vi "edit sensor.vi"(0 "CalibrationData in":T1, 1 "new":bool, 5 "id":u32) -> (4 "CalibrationData out":T1, 6 "canceled":bool, 8 "row":i32)   [LabVIEW 2019, in "GUI Sensor Lib.lvclass"]
uses:
  GUI Sensor Lib.lvclass
  TypeDef/CalibrationData.ctl
  TypeDef/GUI Setting Channel.ctl
  TypeDef/SensorCalibrationData.ctl
panel:
  in  "Scaled":dbl caption="Калиброванное  значение"
  in  "Raw":dbl caption="Необработанное значение"
  in  "ref channel":i16(ring) caption="Канал" items=["Ввод необработанного зачения вручную"=-1]
  in  "data":i32(listbox)
  in  "Remove":bool
  in  "Add":bool
  out "XY Graph - Dark":cluster{dbl[], dbl[]}[](graph)
  in  "Close":bool
  in  "OK":bool
  in  "name":string caption="Название"
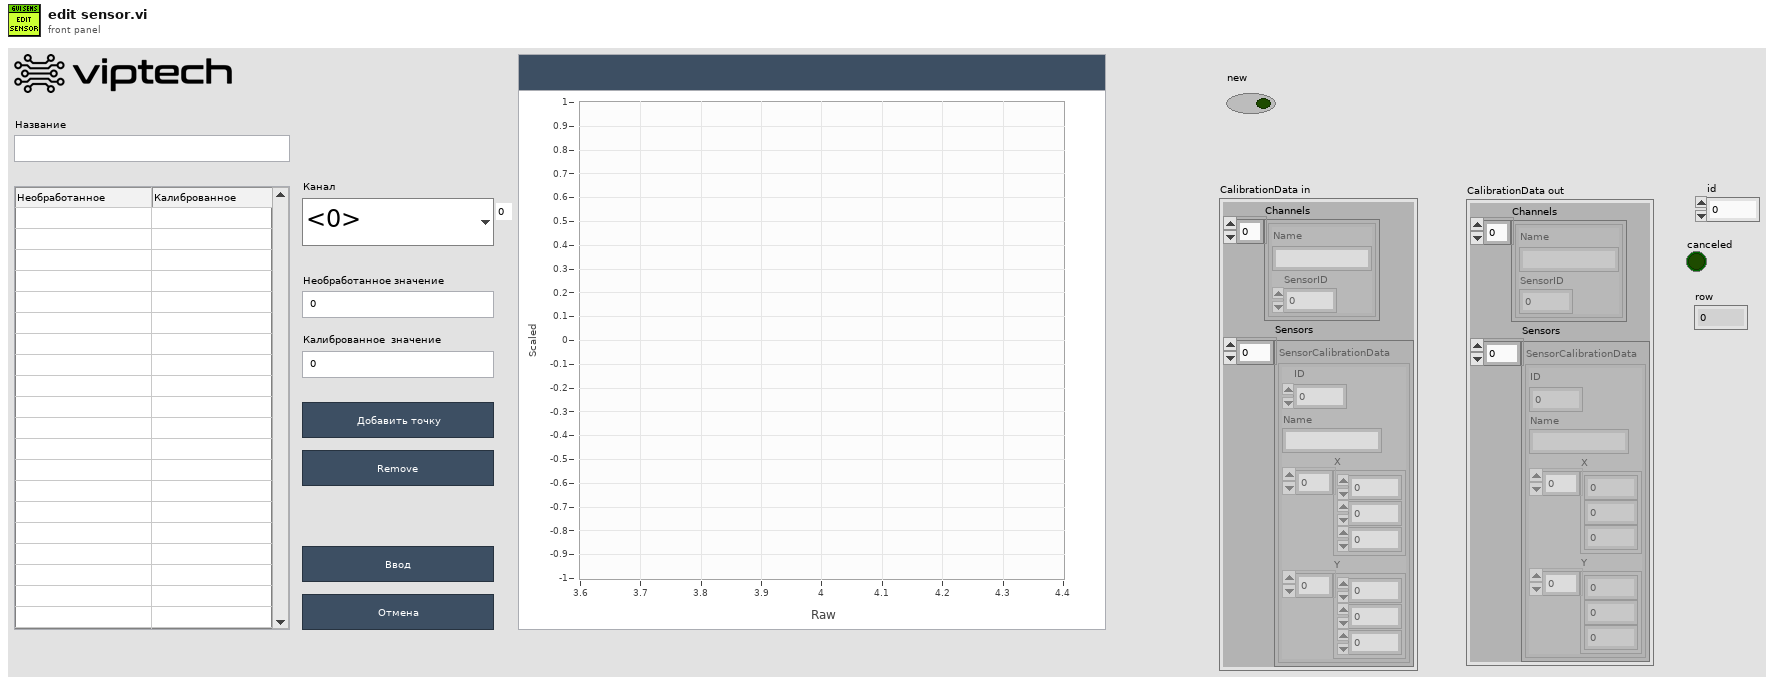
[diagram p1: front panel]
types:
  T1 = typedef "CalibrationData.ctl" = cluster{"Channels":T2[], "Sensors":T3[]}
  T2 = typedef "GUI Setting Channel.ctl" = cluster{"Name":string, "SensorID":u32}
  T3 = typedef "SensorCalibrationData.ctl" = cluster{"ID":u32, "Name":string, "X":dbl[], "Y":dbl[]}
  T4 = enum8{"Enabled", "Disabled", "Disabled and Grayed Out"}
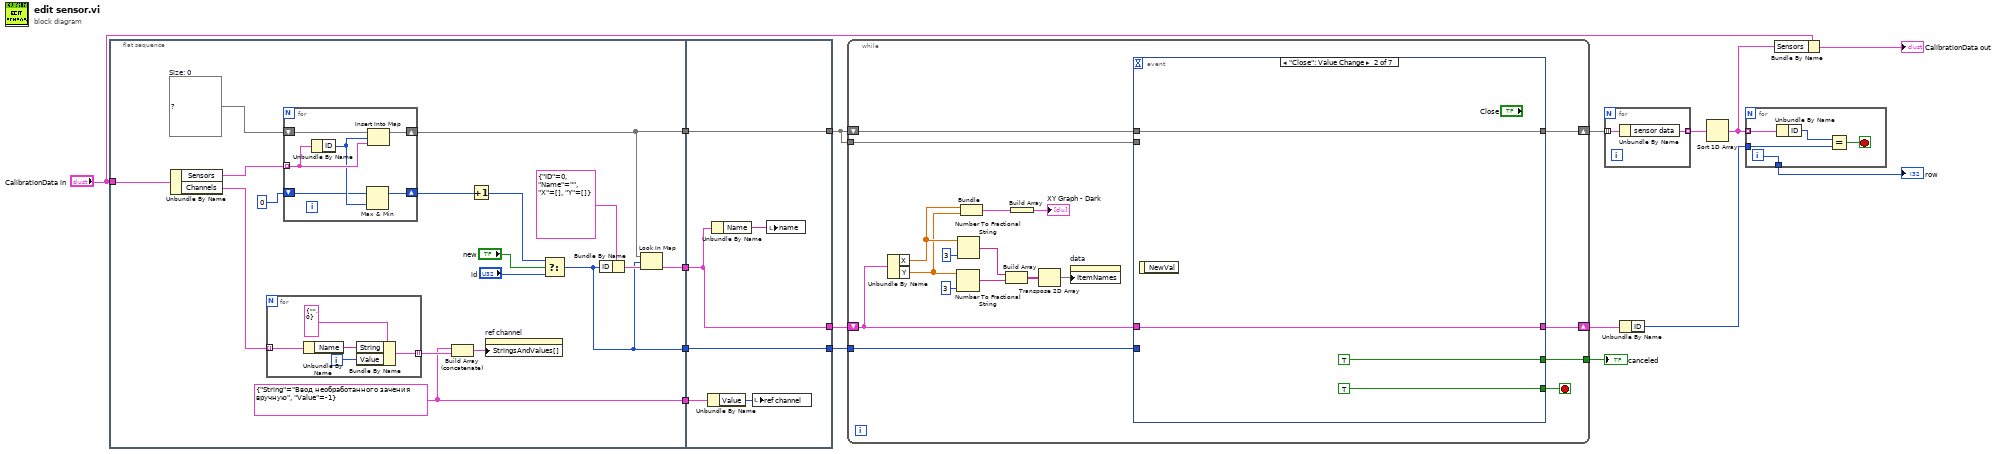
[diagram p0: block diagram]
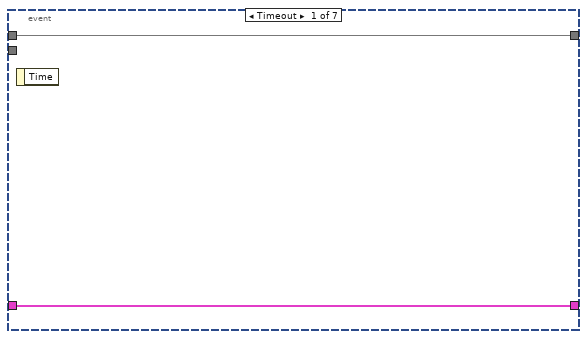
[diagram p2: hidden frame]
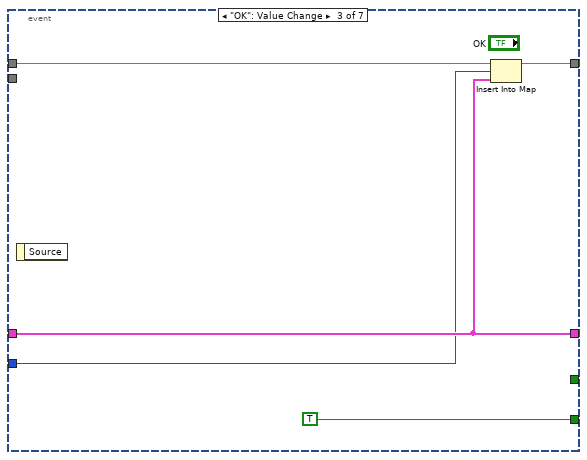
[diagram p3: hidden frame]
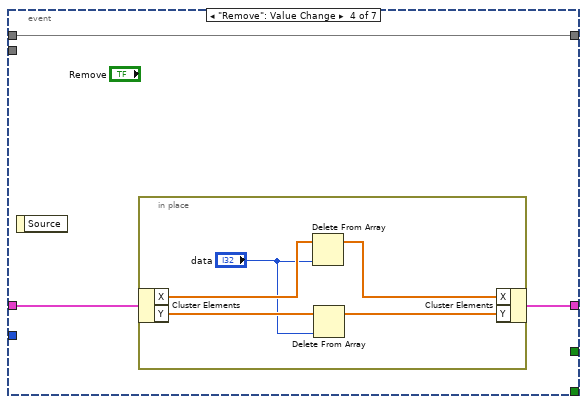
[diagram p4: hidden frame]
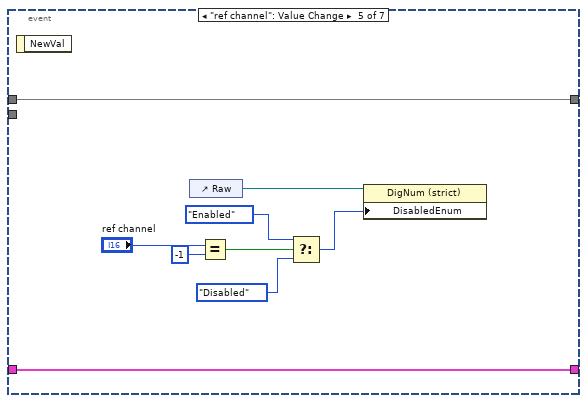
[diagram p5: hidden frame]
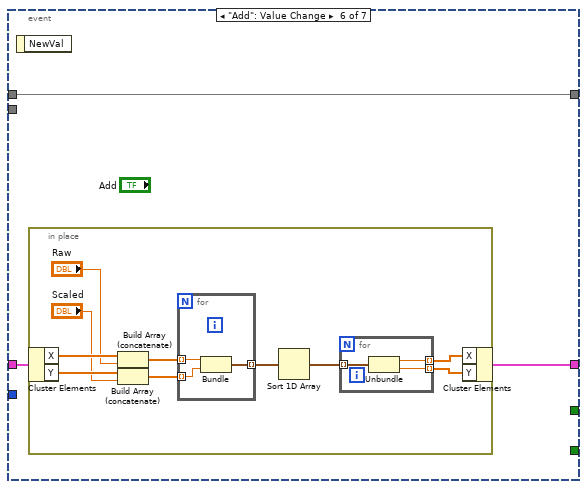
[diagram p6: hidden frame]
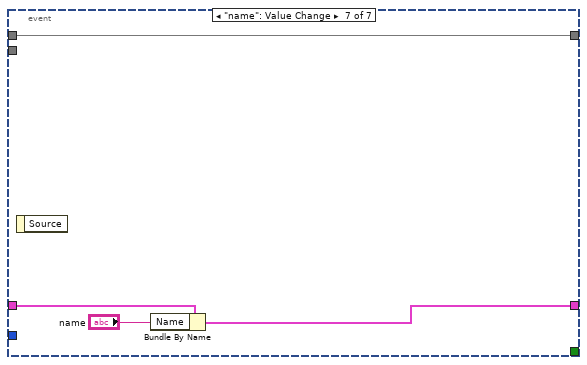
[diagram p7: hidden frame]
diagram:
  n1 = flat-sequence {
    tunnel: [w33] -> w7
    tunnel: [w25] -> w6
    tunnel: [w23] -> w5
    tunnel: [w18] -> w4
    tunnel: "CalibrationData in" -> [w17]
    tunnel: [w49] -> w11
    tunnel: [w45] -> w12
    tunnel: [w50] -> w16
    tunnel: w7 -> [w50]
    tunnel: w6 -> [w45]
    tunnel: w5 -> [w49]
    tunnel: w4 -> [w47]
    frame #0 {
      w18 = cluster{"String":string, "Value":i16} {"String"="Ввод необработанного зачения вручную", "Value"=-1}
      w31 = map{u32, T3} {}  # Size: 0
      n2 = Unbundle By Name(w17) -> ("Sensors"=w22:T3[], "Channels"=w21:T2[])
      n3 = for {
        tunnel: w21 -> [w38] mode=indexing
        tunnel: [w34] -> w20 mode=indexing
        i -> [w36]
        n4 = Unbundle By Name(w38) -> ("Name"=w35:string)
        n5 = Bundle By Name(cluster=cluster{"String":string, "Value":i16} {"String"="", "Value"=0}, "String"=w35, "Value"=w36) -> (w34:cluster{"String":string, "Value":i16})
      }
      n6 = for {
        tunnel: w22 -> [w44] mode=indexing
        shift-right: [w43] -> w33
        shift-left: w31 -> [w42]
        shift-right: [w41] -> w28
        shift-left: u32 0 -> [w39]
        n7 = Unbundle By Name(w44) -> ("ID"=w40:u32)
        n8 = Max & Min(x=w39, y=w40) -> (max(x,y)=w41:u32)  [unwired: 1 out]
        n9 = Insert Into Map(map in=w42, key=w40, value=w44) -> (map out=w43:map{u32, T3})  [unwired: 2 out]
      }
      n10 = Build Array (concatenate)(w18, w20) -> (w19:cluster{"String":string, "Value":i16}[])
      n11 = Increment(x=w28) -> (x+1=w27:u32)
      n12 = property on="ref channel" class="Ring (strict)"("StringsAndValues[]"=w19) -> ()  [unwired: 2 in, 2 out]
      n13 = Select(t=w27, s="new", f="id") -> (s? t:f=w23:u32)
      n14 = Bundle By Name(cluster=T3 {"ID"=0, "Name"="", "X"=[], "Y"=[]} ("sensor data"), "ID"=w23) -> (w24:T3)
      n15 = Look In Map(map=w33, key=w23, default value=w24) -> (value=w25:T3)  [unwired: 1 out]
    }
    frame #1 {
      n16 = Unbundle By Name(w47) -> ("Value"=w48:i16)
      n17 = Unbundle By Name(w45) -> ("Name"=w46:string)
      n18 = local write "ref channel"(w48) -> ()
      n19 = local write "name"(w46) -> ()
    }
  }
  n20 = while {
    shift-right: [w66] -> w14
    shift-left: w16 -> [w67]
    tunnel: w16 -> [w65]
    tunnel: [w64] -> w15
    shift-right: [w63] -> w10
    shift-left: w12 -> [w62]
    tunnel: w11 -> [w61]
    stop <- w68 stop-if-true
    n21 = Unbundle By Name(w62) -> ("X"=w53:dbl[], "Y"=w52:dbl[])
    n22 = Number To Fractional String(number=w52, precision (6)=i16 3) -> (F-format string=w57:string[])  [unwired: 2 in]
    n23 = Number To Fractional String(number=w53, precision (6)=i16 3) -> (F-format string=w58:string[])  [unwired: 2 in]
    n24 = Bundle("X"=w53, "Y"=w52) -> (w55:cluster{"X":dbl[], "Y":dbl[]})  [unwired: 1 in]
    n25 = Build Array(w58, w57) -> (w56:string[][])
    n26 = Build Array(w55) -> (→"XY Graph - Dark":cluster{"X":dbl[], "Y":dbl[]}[])
    n27 = Transpose 2D Array(2D array=w56) -> (transposed array=w51:string[][])
    n28 = property on="data" class="MCListbox (strict)"("ItemNames"=w51) -> ()  [unwired: 2 in, 2 out]
    n29 = event shown="[1] \"Close\": Value Change" {
      selector: _ -> [_ _ _ _ _ _ _]
      dyn-events: _ -> [_ _ _ _ _ _ _]
      timeout: _ -> [_ _ _ _ _ _ _]
      tunnel: [_ TRUE ("Close") TRUE ("Close") _ _ _ _] -> w68
      tunnel: w67 -> [w70 _ w76 w82 w96 w99 w119]
      tunnel: [w70 w74 w77 w82 w96 w99 w119] -> w66
      tunnel: w65 -> [_ w74 _ _ _ _ _]
      tunnel: [_ TRUE _ _ _ _ _] -> w64
      tunnel: w62 -> [w69 w71 w78 w81 w95 w98 w118]
      tunnel: [w69 w71 w78 w80 w95 w97 w117] -> w63
      tunnel: w61 -> [_ _ w75 _ _ _ _]
      event Timeout {
        n30 = event-data() -> ()  [unwired: 1 in, 1 out]
      }
      event "Close": Value Change {
        n31 = event-data() -> ()  [unwired: 1 in, 1 out]
      }
      event "OK": Value Change {
        n32 = event-data() -> ()  [unwired: 1 in, 1 out]
        n33 = Insert Into Map(map in=w76, key=w75, value=w78) -> (map out=w77:map{u32, T3})  [unwired: 2 out]
      }
      event "Remove": Value Change {
        n34 = event-data() -> ()  [unwired: 1 in, 1 out]
        n35 = in-place {
          n36 = in-place-cluster #1(w81) -> ("X"=w87:dbl[], "Y"=w86:dbl[])
          n37 = Delete From Array(array=w87, index="data") -> (array with subset deleted=w84:dbl[])  [unwired: 1 in, 1 out]
          n38 = Delete From Array(array=w86, index="data") -> (array with subset deleted=w85:dbl[])  [unwired: 1 in, 1 out]
          n39 = in-place-cluster #1("X"=w84, "Y"=w85) -> (w80:T3)
        }
      }
      event "ref channel": Value Change {
        n40 = event-data() -> ()  [unwired: 1 in, 1 out]
        n41 = control-ref of="Raw"() -> (w92:refnum<vi>)
        n42 = Equal?(x="ref channel", y=i16 -1) -> (x = y?=w90:bool)
        n43 = Select(t=T4."Enabled" ("Disabled"), s=w90, f=T4."Disabled") -> (s? t:f=w88:T4)
        n44 = property class="DigNum (strict)"(reference=w92, "DisabledEnum"=w88) -> ()  [unwired: 1 in, 2 out]
      }
      event "Add": Value Change {
        n45 = event-data() -> ()  [unwired: 1 in, 1 out]
        n46 = in-place {
          n47 = in-place-cluster #2(w98) -> ("X"=w109:dbl[], "Y"=w108:dbl[])
          n48 = Build Array (concatenate)(w109, "Raw") -> (w103:dbl[])
          n49 = Build Array (concatenate)(w108, "Scaled") -> (w102:dbl[])
          n50 = for {
            tunnel: w103 -> [w115] mode=indexing
            tunnel: w102 -> [w114] mode=indexing
            tunnel: [w113] -> w104 mode=indexing
            n51 = Bundle("Raw"=w115, "Scaled"=w114) -> (w113:cluster{"Raw":dbl, "Scaled":dbl})  [unwired: 1 in]
          }
          n52 = Sort 1D Array(array=w104) -> (sorted array=w105:cluster{"Raw":dbl, "Scaled":dbl}[])
          n53 = for {
            tunnel: w105 -> [w112] mode=indexing
            tunnel: [w111] -> w101 mode=indexing
            tunnel: [w110] -> w100 mode=indexing
            n54 = Unbundle(w112) -> ("Raw"=w111:dbl, "Scaled"=w110:dbl)
          }
          n55 = in-place-cluster #2("X"=w101, "Y"=w100) -> (w97:T3)
        }
      }
      event "name": Value Change {
        n56 = event-data() -> ()  [unwired: 1 in, 1 out]
        n57 = Bundle By Name(cluster=w118, "Name"="name") -> (w117:T3)
      }
    }
  }
  "canceled" <- w15
  n58 = for {
    tunnel: w14 -> [w121] mode=indexing
    tunnel: [w120] -> w13 mode=indexing
    n59 = Unbundle By Name(w121) -> ("sensor data"=w120:T3)
  }
  n60 = Unbundle By Name(w10) -> ("ID"=w9:u32)
  n61 = Sort 1D Array(array=w13) -> (sorted array=w1:T3[])
  n62 = for {
    tunnel: w1 -> [w126] mode=indexing
    tunnel: w9 -> [w124]
    tunnel: [w122] -> w8
    i -> [w122]
    stop <- w123 stop-if-true
    n63 = Unbundle By Name(w126) -> ("ID"=w125:u32)
    n64 = Equal?(x=w125, y=w124) -> (x = y?=w123:bool)
  }
  "row" <- w8
  n65 = Bundle By Name(cluster="CalibrationData in", "Sensors"=w1) -> (→"CalibrationData out":T1)
